vi "Create.vi"(6 "noSignals":i32[](array[numeric]), 7 "Container ID":string, 8 "error in (no error)":errorcluster, 9 "Package Data":T1[](array[typedef]) {"payload" format="%x"; "timestamp" format="%<%.7X\n%x>T"; "type" items=["FlexRay Data"=32, "FlexRay Null"=33, "FlexRay Symbol"=34, "Log Trigger"=225, "Start Trigger"=226]; "cycle count" max=63 step=1}, 10 "Conversion References":refnum<k21>[](array[refnum]), 11 "DataContainer in":refnum<class "DataContainer.lvclass">) -> (0 "error out":errorcluster, 3 "DataContainer out":refnum<class "DataContainer.lvclass">)   [LabVIEW 2023, in "DataContainer.lvclass"]
uses:
  DataContainer.lvclass
  <vilib>/xnet/xnet.llb/XNET Frame FlexRay.ctl
  <vilib>/xnet/xnet.llb/XNET Frame Type FlexRay.ctl
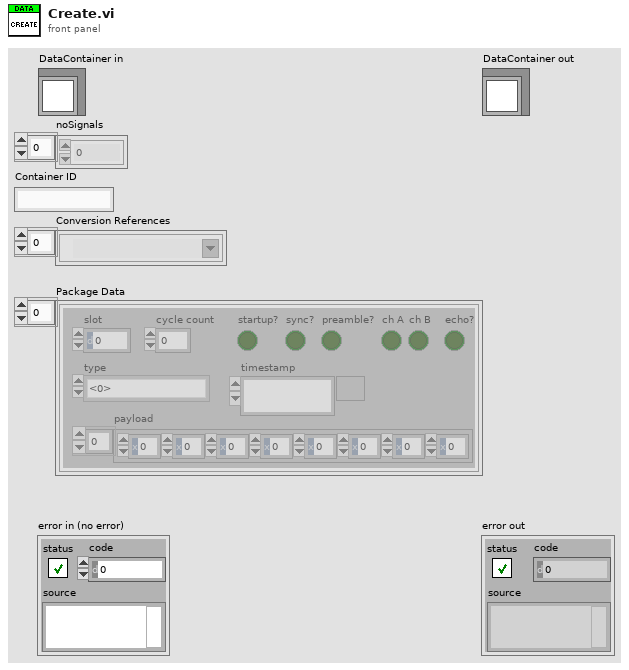
[diagram p1: front panel]
types:
  T1 = typedef "XNET Frame FlexRay.ctl" = cluster{"timestamp":timestamp, "payload":u8[], "slot":u16, "type":T2, "cycle count":u8, "startup?":bool, "sync?":bool, "preamble?":bool, "ch A":bool, "ch B":bool, "echo?":bool}
  T2 = typedef "XNET Frame Type FlexRay.ctl" = u8
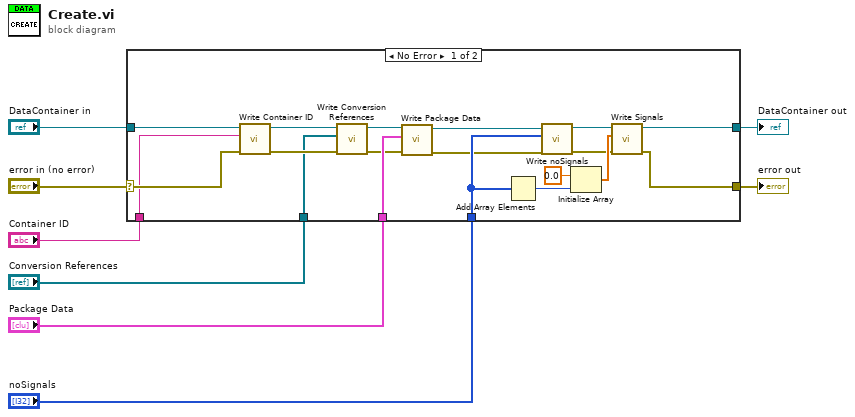
[diagram p0: block diagram]
diagram:
  n1 = case shown="No Error" "error in (no error)" {
    selector: "error in (no error)" -> [w24 w29]
    tunnel: [w22 w29] -> w7
    tunnel: [w25 w28] -> w5
    tunnel: "DataContainer in" -> [w27 w28]
    tunnel: "noSignals" -> [w21 _]
    tunnel: "Container ID" -> [w17 _]
    tunnel: "Conversion References" -> [w16 _]
    tunnel: "Package Data" -> [w15 _]
    frame No Error {
      n2 = call-dynamic "Write Container ID.vi"("error in (no error)"=w24, "Container ID"=w17, "DataContainer in"=w27) -> ("error out"=w23:errorcluster, "DataContainer out"=w26:refnum<class "DataContainer.lvclass">)  [unwired: 7 in]
      n3 = call-dynamic "Write Conversion References.vi"("error in (no error)"=w23, "Conversion References"=w16, "DataContainer in"=w26) -> ("error out"=w11:errorcluster, "DataContainer out"=w12:refnum<class "DataContainer.lvclass">)  [unwired: 7 in]
      n4 = call-dynamic "Write Package Data.vi"("error in (no error)"=w11, "Package Data"=w15, "DataContainer in"=w12) -> ("error out"=w9:errorcluster, "DataContainer out"=w10:refnum<class "DataContainer.lvclass">)  [unwired: 7 in]
      n5 = Add Array Elements(numeric array=w21) -> (sum=w20:i32)
      n6 = call-dynamic "Write noSignals.vi"("error in (no error)"=w9, "noSignals"=w21, "DataContainer in"=w10) -> ("error out"=w13:errorcluster, "DataContainer out"=w14:refnum<class "DataContainer.lvclass">)  [unwired: 7 in]
      n7 = Initialize Array(0.0 ("element"), w20) -> (w18:dbl[])
      n8 = call-dynamic "Write Signals.vi"("error in (no error)"=w13, "Signals"=w18, "DataContainer in"=w14) -> ("error out"=w22:errorcluster, "DataContainer out"=w25:refnum<class "DataContainer.lvclass">)  [unwired: 7 in]
    }
    frame Error {
    }
  }
  "error out" <- w7
  "DataContainer out" <- w5
